vi "Swerve Begin.vi"(8 "Error In":errorcluster) -> (0 "Error Out":errorcluster)   [LabVIEW 2018]
uses:
  <vilib>/Rock Robotics/SystemInterfaces/AI/FPGA_AIChannel.ctl
  <vilib>/Rock Robotics/WPI/ThirdParty/Phoenix-LabVIEW/Motor Controller/Controls/CTRE_Phoenix_MotorControl_NeutralMode.ctl
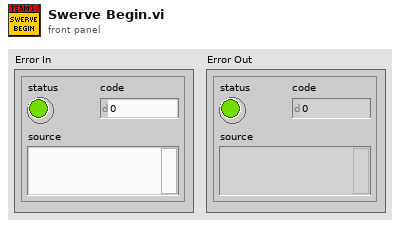
[diagram p1: front panel]
types:
  T1 = typedef "FPGA_AIChannel.ctl" = enum8{"AI 0", "AI 1", "AI 2", "AI 3", "AI MXP 0", "AI MXP 1", "AI MXP 2", "AI MXP 3", "Invalid"}
  T2 = typedef "CTRE_Phoenix_MotorControl_NeutralMode.ctl" = enum8{"EEPROMSetting", "Override to Coast", "Override to Brake"}
  T3 = typedef "WPI_MotorControlDeviceRef.ctl" = cluster{"DeviceStatus":errorcluster, "Type":T4, "PWM":cluster{"PWM Channel":T5, "DeadBand":T6}, "CAN":cluster{"Device Number":u8, "SetOutput VI Ref":variant, "GetOutput VI Ref":variant, "Enable VI Ref":variant, "Disable VI Ref":variant, "Data":variant}, "Invert":bool, "DIO PWM":cluster{"PWM \"Enable\" Channel":T5, "DIOChannel":T7, "PWM Rate":dbl}}
  T4 = typedef "WPI_MotorControlType.ctl" = enum16{"PWM", "CAN", "DIO PWM"}
  T5 = typedef "FPGA_DIOPWMChannel.ctl" = enum8{"PWM 0", "PWM 1", "PWM 2", "PWM 3", "PWM 4", "PWM 5", "PWM 6", "PWM 7", "PWM 8", "PWM 9", "PWM MXP 0", "PWM MXP 1", "PWM MXP 2", "PWM MXP 3", "PWM MXP 4", "PWM MXP 5", "PWM MXP 6", "PWM MXP 7", "PWM MXP 8", "PWM MXP 9", "Invalid"}
  T6 = typedef "WPI_PWMDeadband.ctl" = cluster{"Name":string, "maxPositivePwm":i32, "minPositivePwm":i32, "centerPwm":i32, "maxNegativePwm":i32, "minNegativePwm":i32, "angularRange":u16}
  T7 = typedef "FPGA_DIOChannel.ctl" = enum8{"DIO 0", "DIO 1", "DIO 2", "DIO 3", "DIO 4", "DIO 5", "DIO 6", "DIO 7", "DIO 8", "DIO 9", "DIO MXP 0", "DIO MXP 1", "DIO MXP 2", "DIO MXP 3", "DIO MXP 4", "DIO MXP 5", "DIO MXP 6", "DIO MXP 7", "DIO MXP 8", "DIO MXP 9", "DIO MXP 10", "DIO MXP 11", "DIO MXP 12", "DIO MXP 13", "DIO MXP 14", "DIO MXP 15", "SPI Port CS1", "SPI Port CS2", "SPI Port CS3", "SPI Port MISO", "SPI Port MOSI", "Invalid"}
  T8 = typedef "WPI_AnalogChannelDevRef.ctl" = cluster{"DevStatus":errorcluster, "Analog Channel":T1}
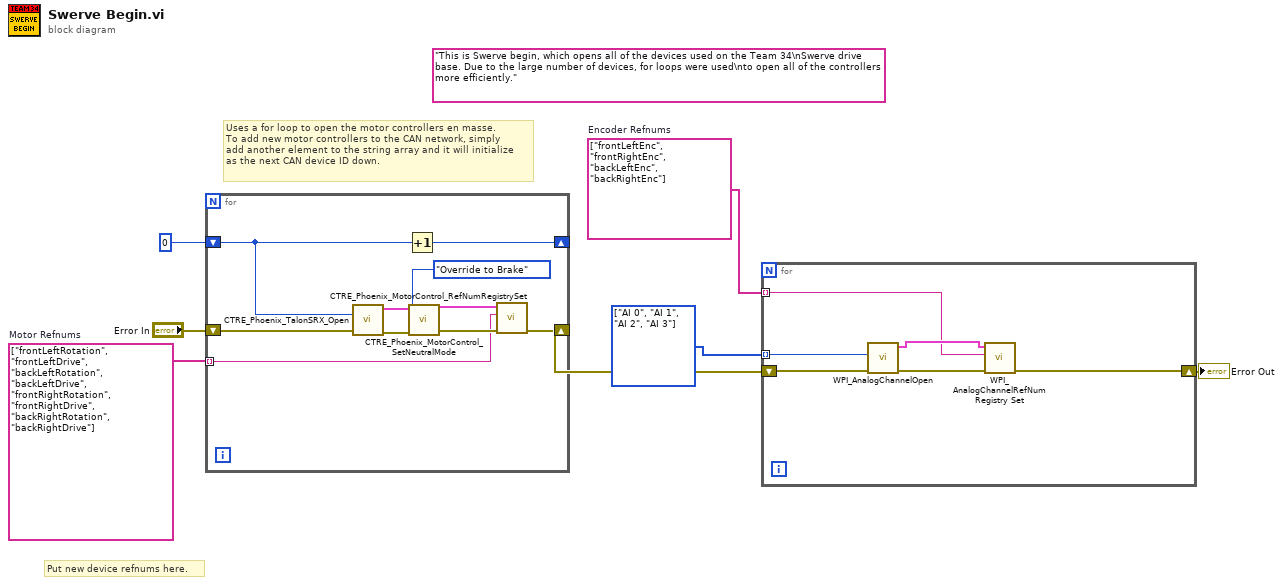
[diagram p0: block diagram]
diagram:
  w1 = T1[] [enum."AI 0", enum."AI 1", enum."AI 2", enum."AI 3"] items=["AI 0", "AI 1", "AI 2", "AI 3", "AI MXP 0", "AI MXP 1", "AI MXP 2", "AI MXP 3", "Invalid"] ("Analog Channel")
  (unwired) "This is Swerve begin, which opens all of the devices used on the Team 34\nSwerve drive base. Due to the large number of devices, for loops were used\nto open all of the controllers more efficiently."
  w5 = string[] ["frontLeftEnc", "frontRightEnc", "backLeftEnc", "backRightEnc"]  # Encoder Refnums
  w6 = string[] ["frontLeftRotation", "frontLeftDrive", "backLeftRotation", "backLeftDrive", "frontRightRotation", "frontRightDrive", "backRightRotation", "backRightDrive"]  # Motor Refnums
  # "Put new device refnums here."
  # "Uses a for loop to open the motor controllers en masse.\nTo add new motor controllers to the CAN network, simply\nadd another element to the string array and it will initialize\nas the next CAN device ID down."
  n1 = for {
    shift-right: [w17] -> _
    shift-left: u8 0 -> [w15]
    tunnel: w6 -> [w9] mode=indexing
    shift-right: [w8] -> w4
    shift-left: "Error In" -> [w16]
    n2 = call <vilib>:"CTRE_Phoenix_TalonSRX_Open.vi"("error in"=w16, "Device Number"=w15) -> ("error out"=w12:errorcluster, "CAN Talon SRX Ref"=w13:T3)  [unwired: 8 in]
    n3 = Increment(x=w15) -> (x+1=w17:u8)
    n4 = call <vilib>:"CTRE_Phoenix_MotorControl_SetNeutralMode.vi"("error in (no error)"=w12, "Motor Control Neutral Mode"=CTRE_Phoenix_MotorControl_NeutralMode."Override to Brake", "PhoenixMotorControlDevRef"=w13) -> ("error out"=w10:errorcluster, "PhoenixMotorControlDevRef"=w11:T3)  [unwired: 7 in]
    n5 = call <vilib>:"CTRE_Phoenix_MotorControl_RefNumRegistrySet.vi"("error in (no error)"=w10, "refnum name"=w9, "PhoenixMotorControlDevRef"=w11) -> ("error out"=w8:errorcluster)  [unwired: 7 in, 1 out]
  }
  n6 = for {
    tunnel: w5 -> [w21] mode=indexing
    shift-right: [w20] -> w2
    shift-left: w4 -> [w18]
    tunnel: w1 -> [w23] mode=indexing
    n7 = call <vilib>:"WPI_AnalogChannelOpen.vi"("error in (no error)"=w18, "Analog Channel"=w23) -> ("error out"=w19:errorcluster, "AIDeviceRef"=w22:T8)  [unwired: 8 in]
    n8 = call <vilib>:"WPI_AnalogChannelRefNum Registry Set.vi"("error in (no error)"=w19, "refnum name"=w21, "AIDeviceRef"=w22) -> ("error out"=w20:errorcluster)  [unwired: 7 in, 1 out]
  }
  "Error Out" <- w2
